vi "Set Matrix Palette Visible.vi"(8 "error in (no error)":errorcluster, 9 "Item Tag":string, 11 "2D Plotmatrix in":refnum<class "XY Plot Matrix.lvclass">) -> (0 "error out":errorcluster, 1 "State Change?":bool, 3 "2D Plotmatrix out":refnum<class "XY Plot Matrix.lvclass">)   [LabVIEW 2017, in "XY Plot Matrix.lvclass"]
uses:
  <vilib>/Math Plots/2D Math Plots/XY Plot Matrix/XY Plot Matrix/XY Plot Matrix.lvclass
  e:/builds/penguin/labview/branches/2017/dev/dist/vi.lib/Math Plots/2D Math Plots/2D Plot/2D Plot/2D Plot.lvclass
  <vilib>/Math Plots/2D Math Plots/2D Plot/2D Plot/2D Plot.lvclass
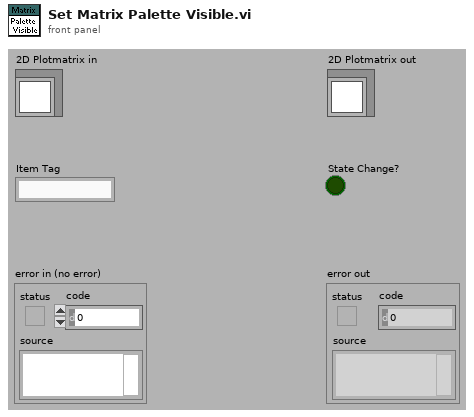
[diagram p1: front panel]
types:
  T1 = typedef "2D Plot.lvclass/Property Cluster.ctl" = cluster{"Graph General":T2, "Format Property":string[], "Scale Array":T3, "Cursor Property":T6, "Annotation List":T8, "Active Cursor":i32, "Active Plot":i32}
  T2 = typedef "2D Plot.lvclass/Graph General Property.ctl" = cluster{"Palette Visible":cluster{"Graph Legend":bool, "Plot Legend":bool, "Auto size":bool, "Number of Plots":u32, "X Scrollbar":bool, "Scale Legend":bool, "Cursor Legend":bool}, "Plot Area Color":cluster{"FG Color":u32, "BG Color":u32}, "Bounds Size":cluster{"Width":u32, "Height":u32}, "Plot Area Bounds":cluster{"Left":i16, "Top":i16, "Right":i16, "Bottom":i16}}
  T3 = typedef "2D Plot.lvclass/Scale Array.ctl" = T4[]
  T4 = typedef "2D Plot.lvclass/Scale Cluster.ctl" = cluster{"General":cluster{"Editable":bool, "Flipped":bool, "Mapping Mode":u8, "Visible":bool, "Style":u8, "Scale Fit":u8}, "Offset and Multiplier":T5, "Range":cluster{"Minimum":dbl, "Maximum":dbl, "Increment":dbl, "Minor Increment":dbl, "Start":dbl}, "Tick Color":cluster{"Major Color":u32, "Minor Color":u32}, "Gird Color":cluster{"Major Color":u32, "Minor Color":u32}, "Marker":cluster{"Visible":bool, "FG Color":u32, "BG Color":u32, "Font Name":string, "Font Size":u32, "Font Bold":bool, "Font Italic":bool, "Font Strikeout":bool, "Font Underline":bool}, "Name Label":cluster{"Visible":bool, "FG Color":u32, "BG Color":u32, "Font Name":string, "Font Size":u32, "Font Bold":bool, "Font Italic":bool, "Font Strikeout":bool, "Font Underline":bool, "Justification":enum16{"Left", "Center", "Right"}, "Text":string}}
  T5 = typedef "LVOffsetAndMultiplierTypeDef.ctl" = cluster{"Offset":dbl, "Multiplier":dbl}
  T6 = typedef "2D Plot.lvclass/Cursor Property.ctl" = cluster{"Cursor List":T7, "Cursor List Addtional":cluster{"Cursor Selection Color":u32, "Line Style":u8, "Line Width":u8, "Visible":bool}[]}
  T7 = typedef "LVCursorListTypeDef.ctl" = cluster{"Name":string, "Color":u32, "Style":u8, "Point Style":u8, "Name Visible":bool, "Allow Drag":bool, "Cursor Mode":u32, "Plot":i32, "Index":i32, "Position":cluster{"X":dbl, "Y":dbl}, "X Scale":u32, "Y Scale":u32, "Watch Plots":i32[], "Watch All Plots":bool, "Plot Area":i32, "Label Offset":cluster{"X":dbl, "Y":dbl}}[]
  T8 = typedef "LVAnnotationListTypeDef.ctl" = cluster{"Name":string, "Color":u32, "Style":u8, "Point Style":u8, "Name Visible":bool, "Allow Drag":bool, "Annotation Mode":u32, "Plot":i32, "Index":i32, "Position":cluster{"X":dbl, "Y":dbl}, "X Scale":u32, "Y Scale":u32, "Show Arrow":bool, "Lock Name":bool, "Plot Area":i32, "Label Offset":cluster{"X":dbl, "Y":dbl}}[]
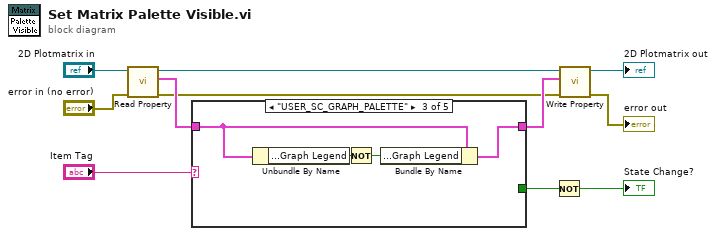
[diagram p0: block diagram]
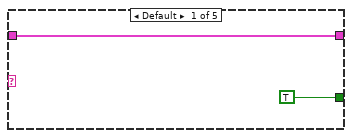
[diagram p2: hidden frame]
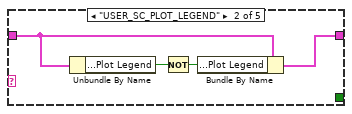
[diagram p3: hidden frame]
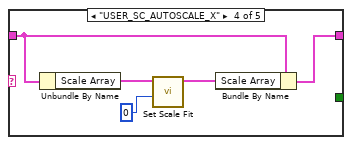
[diagram p4: hidden frame]
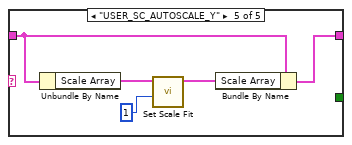
[diagram p5: hidden frame]
diagram:
  n1 = call <vilib>:"Read Property.vi"("error in (no error)"="error in (no error)", "2D Plot.lvclass in"="2D Plotmatrix in") -> ("error out"=w1:errorcluster, "XY Graph Property Cluster"=w8:T1, "2D Plot.lvclass out"=w10:refnum<class "XY Plot Matrix.lvclass">)  [unwired: 7 out]
  n2 = case shown="\"USER_SC_GRAPH_PALETTE\"" "Item Tag" {
    tunnel: w8 -> [w13 w15 w21 w23 w28]
    tunnel: [w13 w14 w20 w22 w27] -> w3
    tunnel: [TRUE _ _ _ _] -> w6
    frame Default {
    }
    frame "USER_SC_PLOT_LEGEND" {
      n3 = Unbundle By Name(w15) -> ("Graph General.Palette Visible.Plot Legend"=w17:bool)
      n4 = Not(x=w17) -> (.not. x?=w16:bool)
      n5 = Bundle By Name(cluster=w15, "Graph General.Palette Visible.Plot Legend"=w16) -> (w14:T1)
    }
    frame "USER_SC_GRAPH_PALETTE" {
      n6 = Unbundle By Name(w21) -> ("Graph General.Palette Visible.Graph Legend"=w19:bool)
      n7 = Not(x=w19) -> (.not. x?=w18:bool)
      n8 = Bundle By Name(cluster=w21, "Graph General.Palette Visible.Graph Legend"=w18) -> (w20:T1)
    }
    frame "USER_SC_AUTOSCALE_X" {
      n9 = Unbundle By Name(w23) -> ("Scale Array"=w26:T3)
      n10 = call <vilib>:"Set Scale Fit.vi"("Axis Index"=0, "Scale Array In"=w26) -> ("Scale Array Out"=w25:T3)  [unwired: 9 out]
      n11 = Bundle By Name(cluster=w23, "Scale Array"=w25) -> (w22:T1)
    }
    frame "USER_SC_AUTOSCALE_Y" {
      n12 = Unbundle By Name(w28) -> ("Scale Array"=w31:T3)
      n13 = call <vilib>:"Set Scale Fit.vi"("Axis Index"=1, "Scale Array In"=w31) -> ("Scale Array Out"=w30:T3)  [unwired: 9 out]
      n14 = Bundle By Name(cluster=w28, "Scale Array"=w30) -> (w27:T1)
    }
  }
  n15 = Not(x=w6) -> (.not. x?=→"State Change?":bool)
  n16 = call <vilib>:"Write Property.vi"("error in (no error)"=w1, "XY Graph Property Cluster"=w3, "2D Plot.lvclass in"=w10) -> ("error out"=→"error out":errorcluster, "2D Plot.lvclass out"=→"2D Plotmatrix out":refnum<class "XY Plot Matrix.lvclass">)  [unwired: 7 out]
